vi "Less Than.vi"(1 "a":string, 2 "b":string) -> (0 "a<b?":bool)   [LabVIEW 2021, in "d13.lvlib"]
uses:
  d13.lvlib
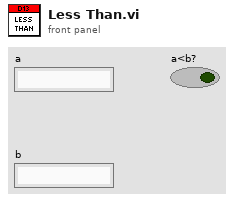
[diagram p1: front panel]
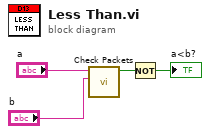
[diagram p0: block diagram]
diagram:
  n1 = call "Check Packets.vi"("Right Packet"="b", "Left Packet"="a") -> ("Correct Order?"=w4:bool)  [unwired: 8 in, 1 out]
  n2 = Not(x=w4) -> (.not. x?=→"a<b?":bool)
